vi "Register Status Change.vi"(0 "CSM Name":string, 1 "TcpRouter-Client in":refnum<class "TcpRouter-Client.lvclass">, 5 "Source CSM Name (* as Default)":string="*", 7 "Status":string, 9 "Response Message (if \"\", same as Source Message)":string, 11 "error in (no error)":errorcluster, 12 "Response Timeout(5000ms)":i32=5000) -> (4 "CSM Name(dup)":string, 15 "error out":errorcluster)   [LabVIEW 2020, in "CSM-TCP-Router.lvlib" / "TcpRouter-Client.lvclass"]
uses:
  TcpRouter-Client.lvclass
  TcpRouter-Client.lvclass/TcpRouter-Client.ctl
  _support/tcp-msg type.ctl
  f32241c3-0036-4787-bc41-e9c1f987f5e1.vi
  <userlib>/_NEVSTOP/Communicable State Machine(CSM)/AdvanceAPI/CSM - Revert Arguments-Safe String.vi
  <userlib>/_NEVSTOP/Communicable State Machine(CSM)/AdvanceAPI/CSM - Keywords.vi
  <userlib>/_NEVSTOP/Communicable State Machine(CSM)/_Polymophic/Build Register Message.vi
  <userlib>/_NEVSTOP/Communicable State Machine(CSM)/_Shared/Trim Single-line Text.vi
  CSM-TCP-Router.lvlib
  <userlib>/_NEVSTOP/Communicable State Machine(CSM)/Communicable State Machine.lvlib
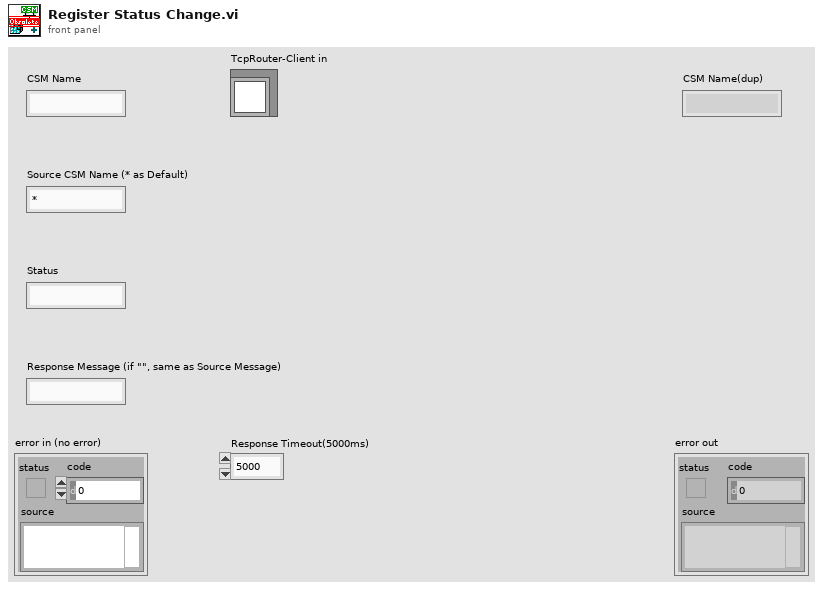
[diagram p1: front panel]
types:
  T1 = typedef "CSM-TCP-Router.lvlib/tcp-msg type.ctl" = enum8{"info", "error", "cmd", "cmd-resp", "resp", "async-resp", "status", "interrupt"}
  T2 = typedef "CSM-TCP-Router.lvlib/TcpRouter-Client.lvclass/Def-TCP-Router REQ-REP.ctl" = cluster{"REQ-REP":refnum<k5>}
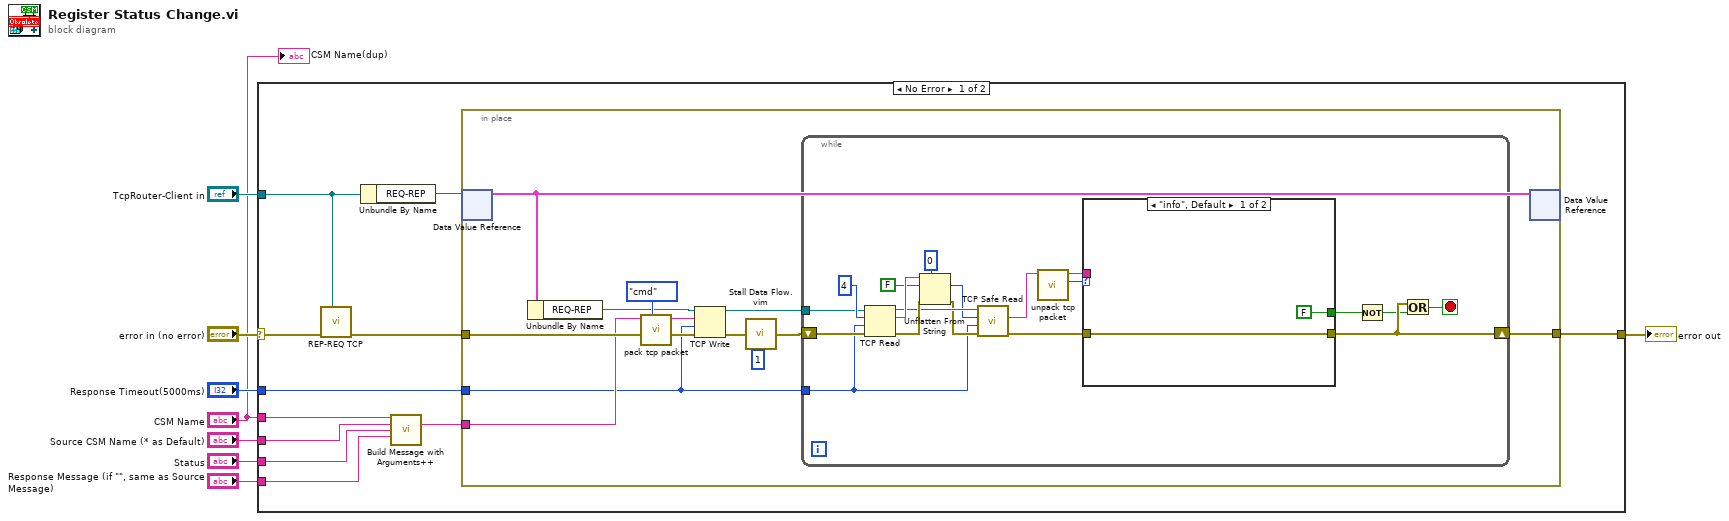
[diagram p0: block diagram]
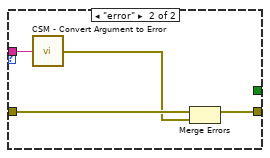
[diagram p2: hidden frame]
diagram:
  n1 = case shown="No Error" "error in (no error)" {
    selector: "error in (no error)" -> [w19 w57]
    tunnel: [w16 w57] -> w7
    tunnel: "TcpRouter-Client in" -> [w14 _]
    tunnel: "Response Timeout(5000ms)" -> [w15 _]
    tunnel: "CSM Name" -> [w11 _]
    tunnel: "Source CSM Name (* as Default)" -> [w12 _]
    tunnel: "Status" -> [w9 _]
    tunnel: "Response Message (if \"\", same as Source Message)" -> [w10 _]
    frame No Error {
      n2 = call "REP-REQ TCP.vi"("TcpRouter-Client in"=w14, "error in (no error)"=w19) -> ("error out"=w18:errorcluster)  [unwired: 7 in, 2 out]
      n3 = Unbundle By Name(w14) -> ("REQ-REP"=w13:refnum<data-value>)
      n4 = call-poly <userlib>:"Build Message with Arguments++.vi"("Target CSM"=w11, "Source CSM (* as Default)"=w12, "Status"=w9, "API (If \"\", Same As \"Status\")"=w10) -> ("CSM Message String"=w17:string)  [unwired: 11 in]
      n5 = in-place {
        in-place-border: w18 -> [w29]
        in-place-border: w17 -> [w28]
        in-place-border: [w23] -> w16
        in-place-border: w15 -> [w22]
        n6 = in-place-dvr #1(w13) -> (w21:T2)  [unwired: 1 out]
        n7 = Unbundle By Name(w21) -> ("REQ-REP"=w20:refnum<k5>)
        n8 = call "pack tcp packet.vi"("tcp-message-type"=tcp-msg_type."cmd", "String"=w28) -> ("TCP Pack"=w31:string)  [unwired: 9 in]
        n9 = TCP Write(connection ID=w20, data in=w31, error in (no error)=w29, 9:w22) -> (connection ID out=w25:refnum<k5>, error out=w27:errorcluster)  [unwired: 1 out]
        n10 = call "Stall Data Flow.vim"("value in"=w27, "milliseconds to wait"=u32 1) -> ("value out"=w24:errorcluster)  [unwired: 1 out]
        n11 = while {
          tunnel: w25 -> [w41]
          shift-right: [w36] -> w23
          shift-left: w24 -> [w40]
          tunnel: w22 -> [w35]
          stop <- w34 stop-if-true
          n12 = TCP Read(connection ID=w41, bytes to read=4, error in (no error)=w40, 9:w35) -> (connection ID out=w48:refnum<k5>, data out=w49:string, error out=w50:errorcluster)  [unwired: 1 in]
          n13 = Unflatten From String(type=0, binary string=w49, data includes array or string size? (T)=FALSE, error in (no error)=w50) -> (value=w46:i32, error out=w45:errorcluster)  [unwired: 2 out]
          n14 = call "TCP Safe Read.vi"("error in (no error)"=w45, "timeout ms (25000)"=w35, "bytes to read"=w46, "TCP Network Connection in"=w48) -> ("error out"=w38:errorcluster, "String"=w47:string)  [unwired: 5 in, 1 out]
          n15 = call "unpack tcp packet.vi"("TCP Pack"=w47) -> ("tcp-message-type"=w39:T1, "String"=w37:string)  [unwired: 9 in]
          n16 = case shown="\"info\", Default" w39 {
            tunnel: w38 -> [w52 w56]
            tunnel: [w52 w54] -> w36
            tunnel: w37 -> [_ w55]
            tunnel: [FALSE _] -> w33
            frame "info", Default {
            }
            frame "error" {
              n17 = call <userlib>:"CSM - Convert Argument to Error.vi"("Argument"=w55) -> ("Error"=w53:errorcluster)  [unwired: 4 in]
              n18 = Merge Errors(w56, w53) -> (w54:errorcluster)
            }
          }
          n19 = Not(x=w33) -> (.not. x?=w32:bool)
          n20 = Or(x=w36, y=w32) -> (x .or. y?=w34:bool)
        }
        n21 = in-place-dvr #1(w21) -> ()  [unwired: 2 out]
      }
    }
    frame Error {
    }
  }
  "error out" <- w7
  "CSM Name(dup)" <- "CSM Name"
